vi "error.vi"(7 "stop":bool, 8 "idx":i32, 11 "Qube":refnum<class "System.lvclass">) -> (0 "abort?":bool, 3 "Qube":refnum<class "System.lvclass">)   [LabVIEW 2021, in "System.lvclass"]
uses:
  System.lvclass
  System.lvclass/System.ctl
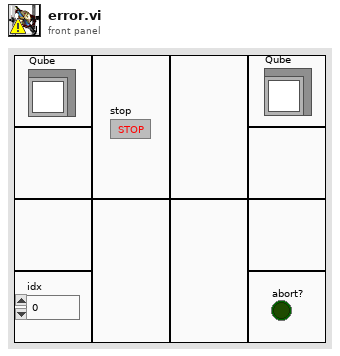
[diagram p1: front panel]
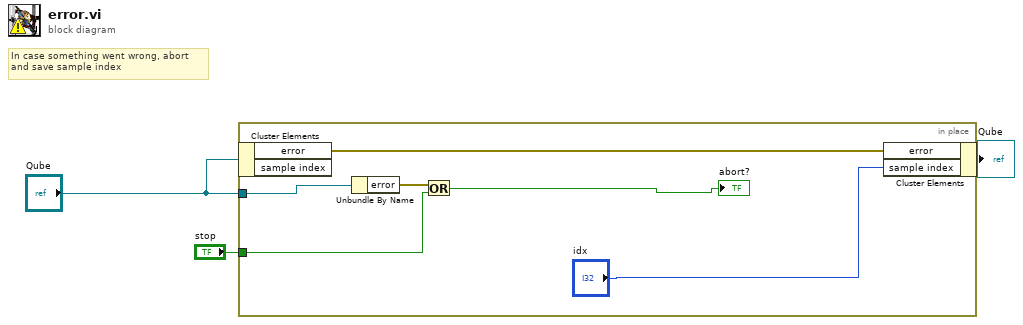
[diagram p0: block diagram]
diagram:
  # "In case something went wrong, abort\nand save sample index"
  n1 = in-place {
    in-place-border: "stop" -> [w7]
    in-place-border: "Qube" -> [w6]
    n2 = in-place-cluster #1("Qube") -> ("error"=w9:errorcluster)  [unwired: 1 out]
    n3 = Unbundle By Name(w6) -> ("error"=w8:errorcluster)
    n4 = Or(x=w8, y=w7) -> (x .or. y?=→"abort?":bool)
    n5 = in-place-cluster #1("error"=w9, "sample index"="idx") -> (→"Qube":refnum<class "System.lvclass">)
  }
